vi "Handle Request.vi"(7 "Processing In":refnum<class "Processing.lvclass">, 11 "WebSocket Handler in":refnum<class "WebSocket Handler.lvclass">) -> (0 "error out":errorcluster, 5 "Processing":refnum<class "Processing.lvclass">)   [LabVIEW 2020, in "HTTP Server.lvlib" / "WebSocket Handler.lvclass"]
uses:
  WebSocket Handler.lvclass
  WebSocket Handler.lvclass/WebSocket Handler.ctl
  Processing/Processing.lvclass
  WebSocket Client/WebSocket Client.lvclass
  WebSocketUpgradeResponse/WebSocketUpgradeResponse.lvclass
  C:/dev/lv20CE/relink/lv-http-util/HTTP Utils/Response/Response.lvclass
  C:/dev/lv20CE/relink/lv-http-server/HTTP Server/WebSocketUpgradeResponse/WebSocketUpgradeResponse.lvclass
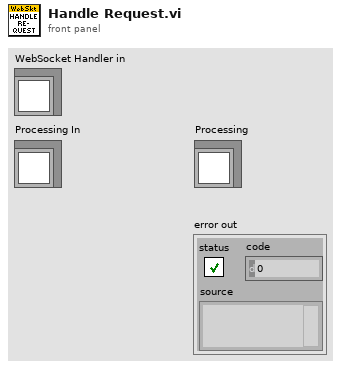
[diagram p1: front panel]
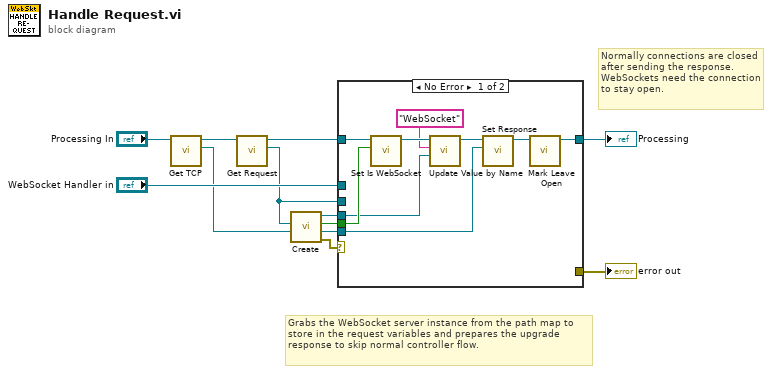
[diagram p0: block diagram]
diagram:
  # "Normally connections are closed after sending the response. WebSockets need the connection to stay open."
  # "Grabs the WebSocket server instance from the path map to store in the request variables and prepares the upgrade response to skip normal controller flow."
  n1 = call "Get TCP.vi"("Processing in"="Processing In") -> ("TCP"=w5:refnum<k5>, "Processing out"=w7:refnum<class "Processing.lvclass">)  [unwired: 9 in]
  n2 = call "Get Request.vi"("Processing in"=w7) -> ("Request"=w6:refnum<class "Request.lvclass">, "Processing out"=w9:refnum<class "Processing.lvclass">)  [unwired: 9 in]
  n3 = call "Create.vi"("TCP"=w5, "Request"=w6) -> ("error out"=w4:errorcluster, "Response out"=w2:refnum<class "WebSocketUpgradeResponse.lvclass">, "Is WS Upgrade"=w3:bool, "WebSocket Client out"=w1:refnum<class "WebSocket Client.lvclass">)  [unwired: 6 in]
  n4 = case shown="No Error" w4 {
    selector: w4 -> [_ w24]
    tunnel: w6 -> [_ _]
    tunnel: [w21 w25] -> w12
    tunnel: [_ w22] -> w11
    tunnel: w9 -> [w20 w25]
    tunnel: "WebSocket Handler in" -> [_ _]
    tunnel: w3 -> [w18 w23]
    tunnel: w2 -> [w13 _]
    tunnel: w1 -> [w14 _]
    frame No Error {
      n5 = call "Set Is WebSocket.vi"("Is WebSocket"=w18, "Processing in"=w20) -> ("Processing out"=w19:refnum<class "Processing.lvclass">)  [unwired: 9 in]
      n6 = call "Update Value by Name.vi"("Value"=w14, "Name"="WebSocket" ("Name / Service / Object"), "Processing in"=w19) -> ("Processing out"=w16:refnum<class "Processing.lvclass">)  [unwired: 7 in, 1 out]
      n7 = call "Set Response.vi"("Response"=w13, "Processing in"=w16) -> ("Processing out"=w17:refnum<class "Processing.lvclass">)  [unwired: 9 in]
      n8 = call "Mark Leave Open.vi"("Processing in"=w17) -> ("Processing out"=w21:refnum<class "Processing.lvclass">)  [unwired: 10 in]
    }
    frame Error {
      n9 = case shown="False" w23 {
        tunnel: w24 -> [_ w26]
        tunnel: [_ w26] -> w22
        frame False {
          # "Not an upgrade request, ignore error."
        }
        frame True {
        }
      }
    }
  }
  "error out" <- w11
  "Processing" <- w12
